vi "Facade.vi"(0 "Data In":T4, 2 "Display State In":T2, 3 "Container State":T3) -> (6 "Data Out":T4, 7 "Display State Out":T2, 8 "Action":T1)   [LabVIEW 2020, in "KColorSliders.xctl"]
uses:
  KColorSliders.xctl
  Data.vi
  <vilib>/_xctls/Container State.ctl
  State.vi
  <vilib>/_xctls/Action.ctl
  <vilib>/_xctls/XControlSupport.lvlib
panel:
  in  "Blue":u8(slide) scale=0.0..255.0
  in  "Green":u8(slide) scale=0.0..255.0
  in  "Red":u8(slide) scale=0.0..255.0
  in  "Color Box":u32(colorbox)
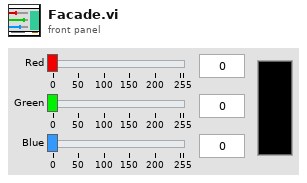
[diagram p1: front panel]
types:
  T1 = typedef "XControlSupport.lvlib/Action.ctl" = cluster{"Data Changed?":bool, "State Changed?":bool, "Action Name":string}
  T2 = typedef "KColorSliders.xctl/State.vi" = cluster{"Numeric":dbl}
  T3 = typedef "XControlSupport.lvlib/Container State.ctl" = cluster{"Indicator?":bool, "Run Mode?":bool, " Refnum":refnum<vi>}
  T4 = typedef "KColorSliders.xctl/Data.vi" = u32
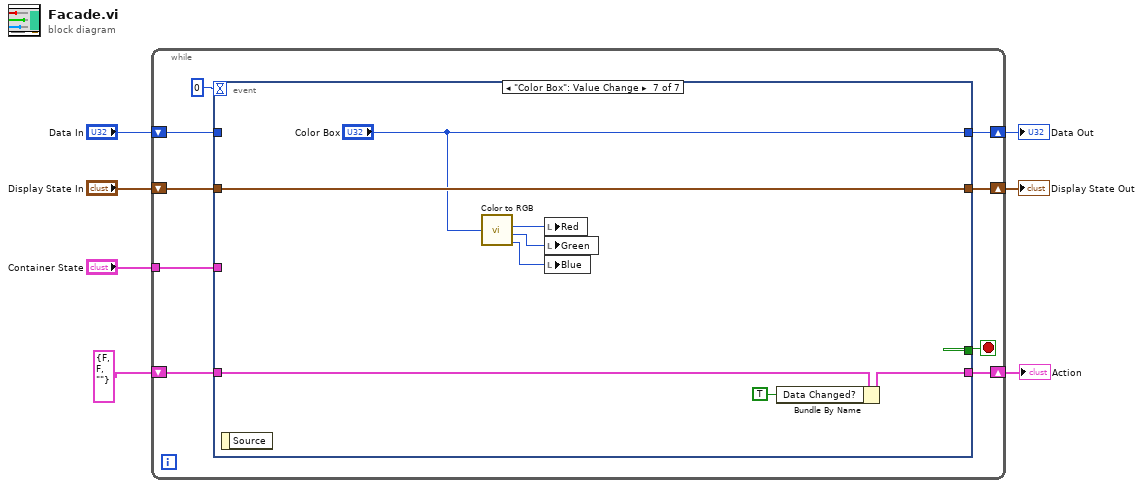
[diagram p0: block diagram]
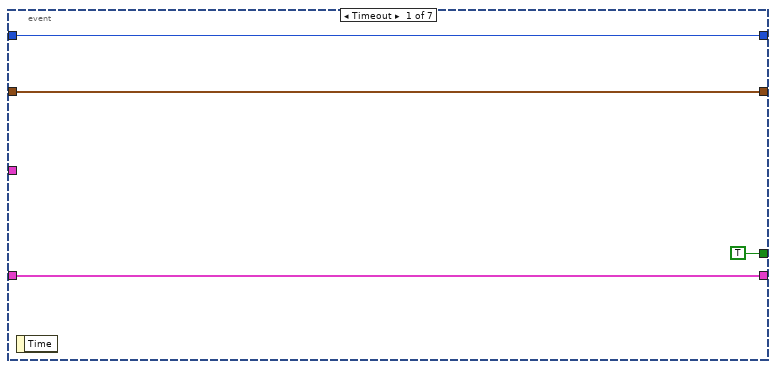
[diagram p2: hidden frame]
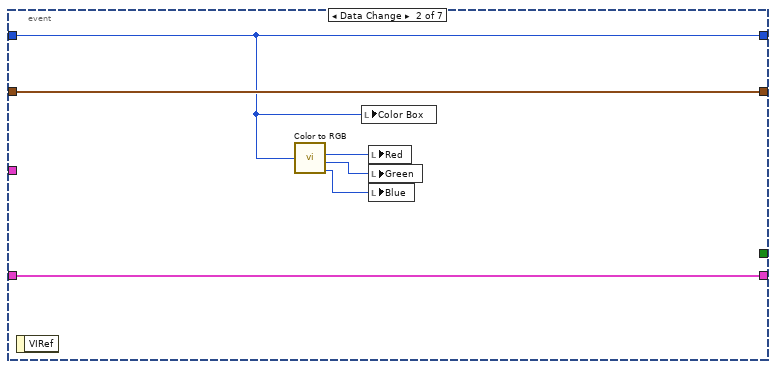
[diagram p3: hidden frame]
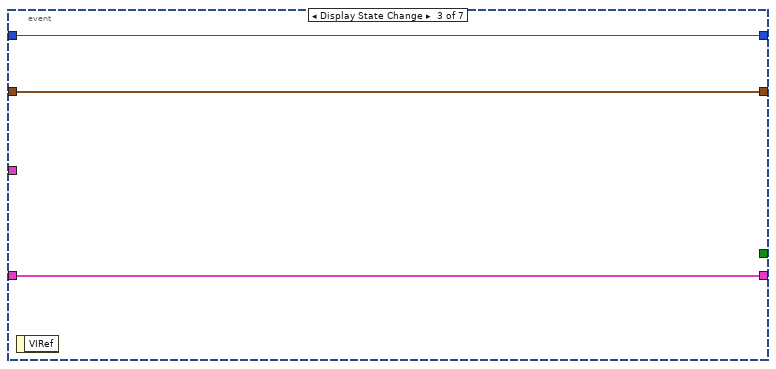
[diagram p4: hidden frame]
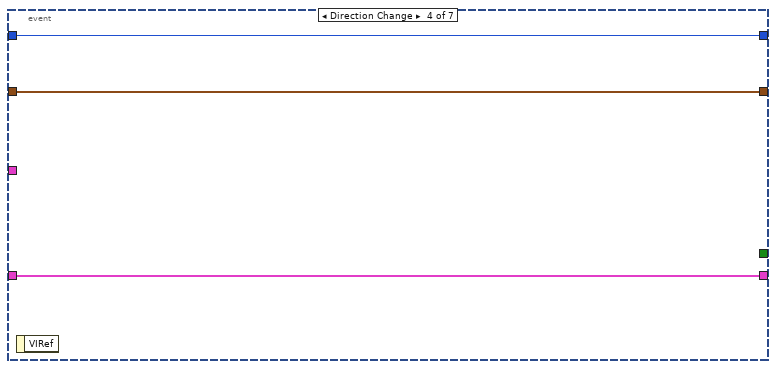
[diagram p5: hidden frame]
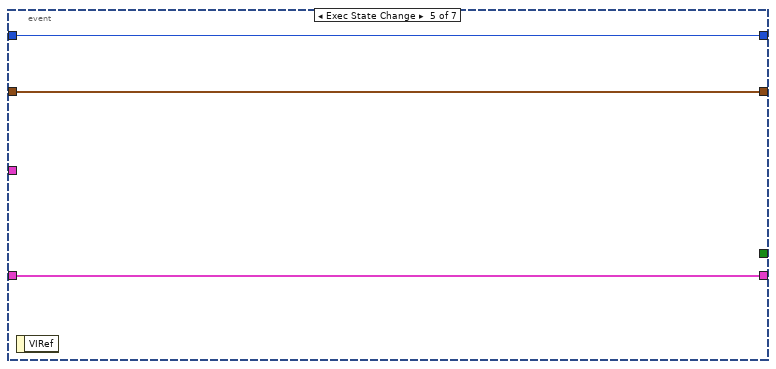
[diagram p6: hidden frame]
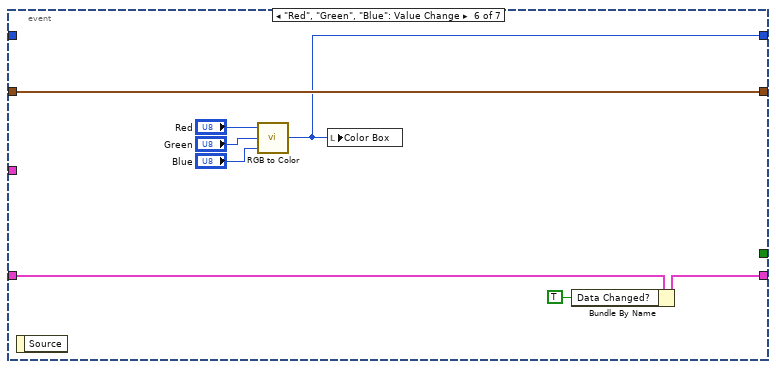
[diagram p7: hidden frame]
diagram:
  n1 = while {
    shift-right: [w15] -> w4
    shift-left: "Display State In" -> [w16]
    tunnel: "Container State" -> [w12]
    shift-right: [w10] -> w7
    shift-left: "Data In" -> [w11]
    shift-right: [w8] -> w2
    shift-left: T1 {"Data Changed?"=FALSE, "State Changed?"=FALSE, "Action Name"=""} ("Action") -> [w9]
    stop <- w14 stop-if-true
    n2 = event shown="[6] \"Color Box\": Value Change" {
      selector: _ -> [_ _ _ _ _ _ _]
      dyn-events: _ -> [_ _ _ _ _ _ _]
      timeout: 0 -> [_ _ _ _ _ _ _]
      tunnel: w16 -> [w18 w26 w29 w32 w35 w43 w51]
      tunnel: [w18 w26 w29 w32 w35 w43 w51] -> w15
      tunnel: [TRUE _ _ _ _ _ _] -> w14
      tunnel: w12 -> [_ _ _ _ _ _ _]
      tunnel: w11 -> [w17 w24 w28 w31 w34 _ _]
      tunnel: [w17 w24 w28 w31 w34 w36 "Color Box"] -> w10
      tunnel: [w19 w25 w27 w30 w33 w41 w49] -> w8
      tunnel: w9 -> [w19 w25 w27 w30 w33 w42 w50]
      event Timeout {
        n3 = event-data() -> ()  [unwired: 1 in, 1 out]
      }
      event Data Change {
        n4 = event-data() -> ()  [unwired: 1 in, 1 out]
        n5 = call <vilib>:"Color to RGB.vi"("Color"=w24) -> ("R"=w23:u8, "G"=w22:u8, "B"=w21:u8)  [unwired: 1 out]
        n6 = local write "Color Box"(w24) -> ()
        n7 = local write "Red"(w23) -> ()
        n8 = local write "Green"(w22) -> ()
        n9 = local write "Blue"(w21) -> ()
      }
      event Display State Change {
        n10 = event-data() -> ()  [unwired: 1 in, 1 out]
      }
      event Direction Change {
        n11 = event-data() -> ()  [unwired: 1 in, 1 out]
      }
      event Exec State Change {
        n12 = event-data() -> ()  [unwired: 1 in, 1 out]
      }
      event "Red", "Green", "Blue": Value Change {
        n13 = event-data() -> ()  [unwired: 1 in, 1 out]
        n14 = call <vilib>:"RGB to Color.vi"("B"="Blue", "G"="Green", "R"="Red") -> ("Color"=w36:u32)
        n15 = local write "Color Box"(w36) -> ()
        n16 = Bundle By Name(cluster=w42, "Data Changed?"=TRUE) -> (w41:T1)
      }
      event "Color Box": Value Change {
        n17 = event-data() -> ()  [unwired: 1 in, 1 out]
        n18 = call <vilib>:"Color to RGB.vi"("Color"="Color Box") -> ("R"=w46:u8, "G"=w45:u8, "B"=w44:u8)  [unwired: 1 out]
        n19 = local write "Red"(w46) -> ()
        n20 = local write "Green"(w45) -> ()
        n21 = local write "Blue"(w44) -> ()
        n22 = Bundle By Name(cluster=w50, "Data Changed?"=TRUE) -> (w49:T1)
      }
    }
  }
  "Display State Out" <- w4
  "Data Out" <- w7
  "Action" <- w2
